vi "FailureDescription.vi"(8 "error in (no error)":errorcluster, 10 "Actual":variant, 11 "Error in":refnum<class "Error.lvclass">) -> (0 "error out":errorcluster, 2 "Failure Description":string, 3 "Error out":refnum<class "Error.lvclass">)   [LabVIEW 2017, in "Transparent Assertions.lvlib" / "Error.lvclass"]
doc: "Return the second part of the scentence \"Failed asserting that ...\""
uses:
  Error.lvclass
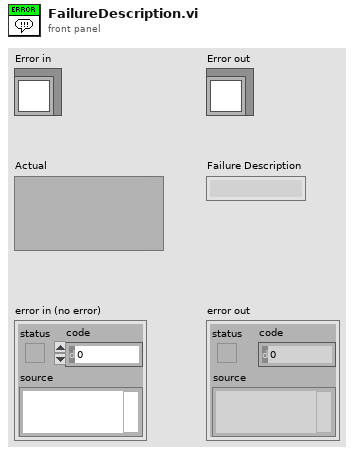
[diagram p1: front panel]
types:
  T1 = typedef "Transparent Assertions.lvlib/Error.lvclass/ErrorType.ctl" = enum16{"error", "warning", "no error"}
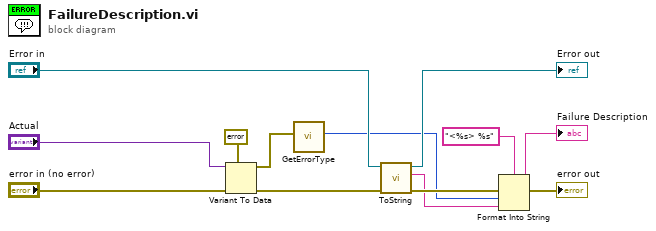
[diagram p0: block diagram]
diagram:
  n1 = Variant To Data(error in="error in (no error)", type=errorcluster {"status"=FALSE, "code"=0, "source"=""} ("error constant"), Variant="Actual") -> (data=w6:errorcluster, error out=w12:errorcluster)
  n2 = call "GetErrorType.vi"("error in (no error)"=w6) -> ("ErrorType"=w1:T1)  [unwired: 10 in]
  n3 = call-dynamic "ToString.vi"("error in (no error)"=w12, "Error in"="Error in") -> ("error out"=w9:errorcluster, "String"=w3:string, "Error out"=→"Error out":refnum<class "Error.lvclass">)  [unwired: 7 in]
  n4 = Format Into String(format string="<%s> %s", error in=w9, w1, w3) -> (resulting string=→"Failure Description":string, error out=→"error out":errorcluster)  [unwired: 1 in]
